vi "Settings Dialog.vi"(8 "error in (no error)":errorcluster, 11 "Settings in":T1={"Hardware Configuration"={"DAQmx Channel 1"="", "DAQmx Channel 2"="", "DAQmx Channel 3"="", "Channel 1 Name"="", "Channel 2 Name"="", "Channel 3 Name"="", "Input Config Channel 1"=-1, "Input Config Channel 2"=-1, "Input Config Channel 3"=-1, "Offset Channel 1"=0.0, "Offset Channel 2"=0.0, "Offset Channel 3"=0.0, "Scale Channel 1"=0.0, "Scale Channel 2"=0.0, "Scale Channel 3"=0.0, "Sample time"=0, "Samples per second"=0.0, "Sample mode"=0, "Samples per channel"=0, "DAQmx AI Task"="", "DAQmx Channel 4"="", "Channel 3 Name 2"="", "Input Config Channel 4"=-1, "Offset Channel 4"=0.0, "Scale Channel 4"=0.0}, "Logging Configuration"={"Log File Base Path"=path "", "TDMS File Reference"=refnum}} {"Hardware Configuration"."Input Config Channel 4" items=["Default"=-1, "RSE"=10083, "NRSE"=10078, "Differential"=10106, "Pseudodifferential"=12529]; "Hardware Configuration"."Input Config Channel 3" items=["Default"=-1, "RSE"=10083, "NRSE"=10078, "Differential"=10106, "Pseudodifferential"=12529]; "Hardware Configuration"."Input Config Channel 2" items=["Default"=-1, "RSE"=10083, "NRSE"=10078, "Differential"=10106, "Pseudodifferential"=12529]; "Hardware Configuration"."Input Config Channel 1" items=["Default"=-1, "RSE"=10083, "NRSE"=10078, "Differential"=10106, "Pseudodifferential"=12529]; "Hardware Configuration"."Sample mode" items=["Hardware Timed Single Point"=12522, "Finite Samples"=10178, "Continuous Samples"=10123]}) -> (0 "error out":errorcluster, 1 "Cancelled?":bool, 2 "UI Refresh Needed?":bool, 3 "Settings out":T1={"Hardware Configuration"={"DAQmx Channel 1"="", "DAQmx Channel 2"="", "DAQmx Channel 3"="", "Channel 1 Name"="", "Channel 2 Name"="", "Channel 3 Name"="", "Input Config Channel 1"=-1, "Input Config Channel 2"=-1, "Input Config Channel 3"=-1, "Offset Channel 1"=0.0, "Offset Channel 2"=0.0, "Offset Channel 3"=0.0, "Scale Channel 1"=0.0, "Scale Channel 2"=0.0, "Scale Channel 3"=0.0, "Sample time"=0, "Samples per second"=0.0, "Sample mode"=0, "Samples per channel"=0, "DAQmx AI Task"="", "DAQmx Channel 4"="", "Channel 3 Name 2"="", "Input Config Channel 4"=-1, "Offset Channel 4"=0.0, "Scale Channel 4"=0.0}, "Logging Configuration"={"Log File Base Path"=path "", "TDMS File Reference"=refnum}} {"Hardware Configuration"."Input Config Channel 4" items=["Default"=-1, "RSE"=10083, "NRSE"=10078, "Differential"=10106, "Pseudodifferential"=12529]; "Hardware Configuration"."Input Config Channel 3" items=["Default"=-1, "RSE"=10083, "NRSE"=10078, "Differential"=10106, "Pseudodifferential"=12529]; "Hardware Configuration"."Input Config Channel 2" items=["Default"=-1, "RSE"=10083, "NRSE"=10078, "Differential"=10106, "Pseudodifferential"=12529]; "Hardware Configuration"."Input Config Channel 1" items=["Default"=-1, "RSE"=10083, "NRSE"=10078, "Differential"=10106, "Pseudodifferential"=12529]; "Hardware Configuration"."Sample mode" items=["Hardware Timed Single Point"=12522, "Finite Samples"=10178, "Continuous Samples"=10123]})   [LabVIEW 2018, in "Settings.lvlib"]
doc: "Dialog for selecting user specified settings."
uses:
  Settings.lvlib
  Settings.ctl
  Acquisition/Hardware Configuration.ctl
  Logging/Logging Configuration.ctl
  <vilib>/Utility/xml.llb/Write to XML File(string).vi
  Acquisition/Acquisition.lvlib
  Logging/Logging.lvlib
panel:
  in  "Scale Channel 4":dbl
  in  "Offset Channel 4":dbl
  in  "Input Config Channel 4":i32(ring)=-1 items=["Default"=-1, "RSE"=10083, "NRSE"=10078, "Differential"=10106, "Pseudodifferential"=12529]
  in  "Input Config Channel 3":i32(ring)=-1 items=["Default"=-1, "RSE"=10083, "NRSE"=10078, "Differential"=10106, "Pseudodifferential"=12529]
  in  "Input Config Channel 2":i32(ring)=-1 items=["Default"=-1, "RSE"=10083, "NRSE"=10078, "Differential"=10106, "Pseudodifferential"=12529]
  in  "Input Config Channel 1":i32(ring)=-1 items=["Default"=-1, "RSE"=10083, "NRSE"=10078, "Differential"=10106, "Pseudodifferential"=12529]
  in  "Channel 4":tag="SimDev1/ai0"
  in  "Channel 4 Name":string="Battery Voltage"
  in  "Scale Channel 3":dbl
  in  "Scale Channel 2":dbl
  in  "Scale Channel 1":dbl
  in  "Offset Channel 3":dbl
  in  "Offset Channel 2":dbl
  in  "Offset Channel 1":dbl
  in  "Sample Mode":u16(ring)=10123 items=["Finite Samples"=10178, "Continuous Samples"=10123, "Hardware Timed Single Point"=12522]
  in  "Samples per channel":u32
  in  "Samples per second":dbl=1000.0
  in  "Sample time in ms":u32=10
  in  "Channel 3 Name":string="Brake torque"
  in  "Channel 2 Name":string="Battery Current"
  in  "Channel 1 Name":string="Battery Voltage"
  in  "Channel 3":tag="SimDev1/ai2"
  in  "Channel 2":tag="SimDev1/ai1"
  in  "Log File Path":path
  in  "Channel 1":tag="SimDev1/ai0"
  in  "Cancel Button":bool
  in  "OK Button":bool
  # "Non visible portion of dialog (needed for connector pane)."
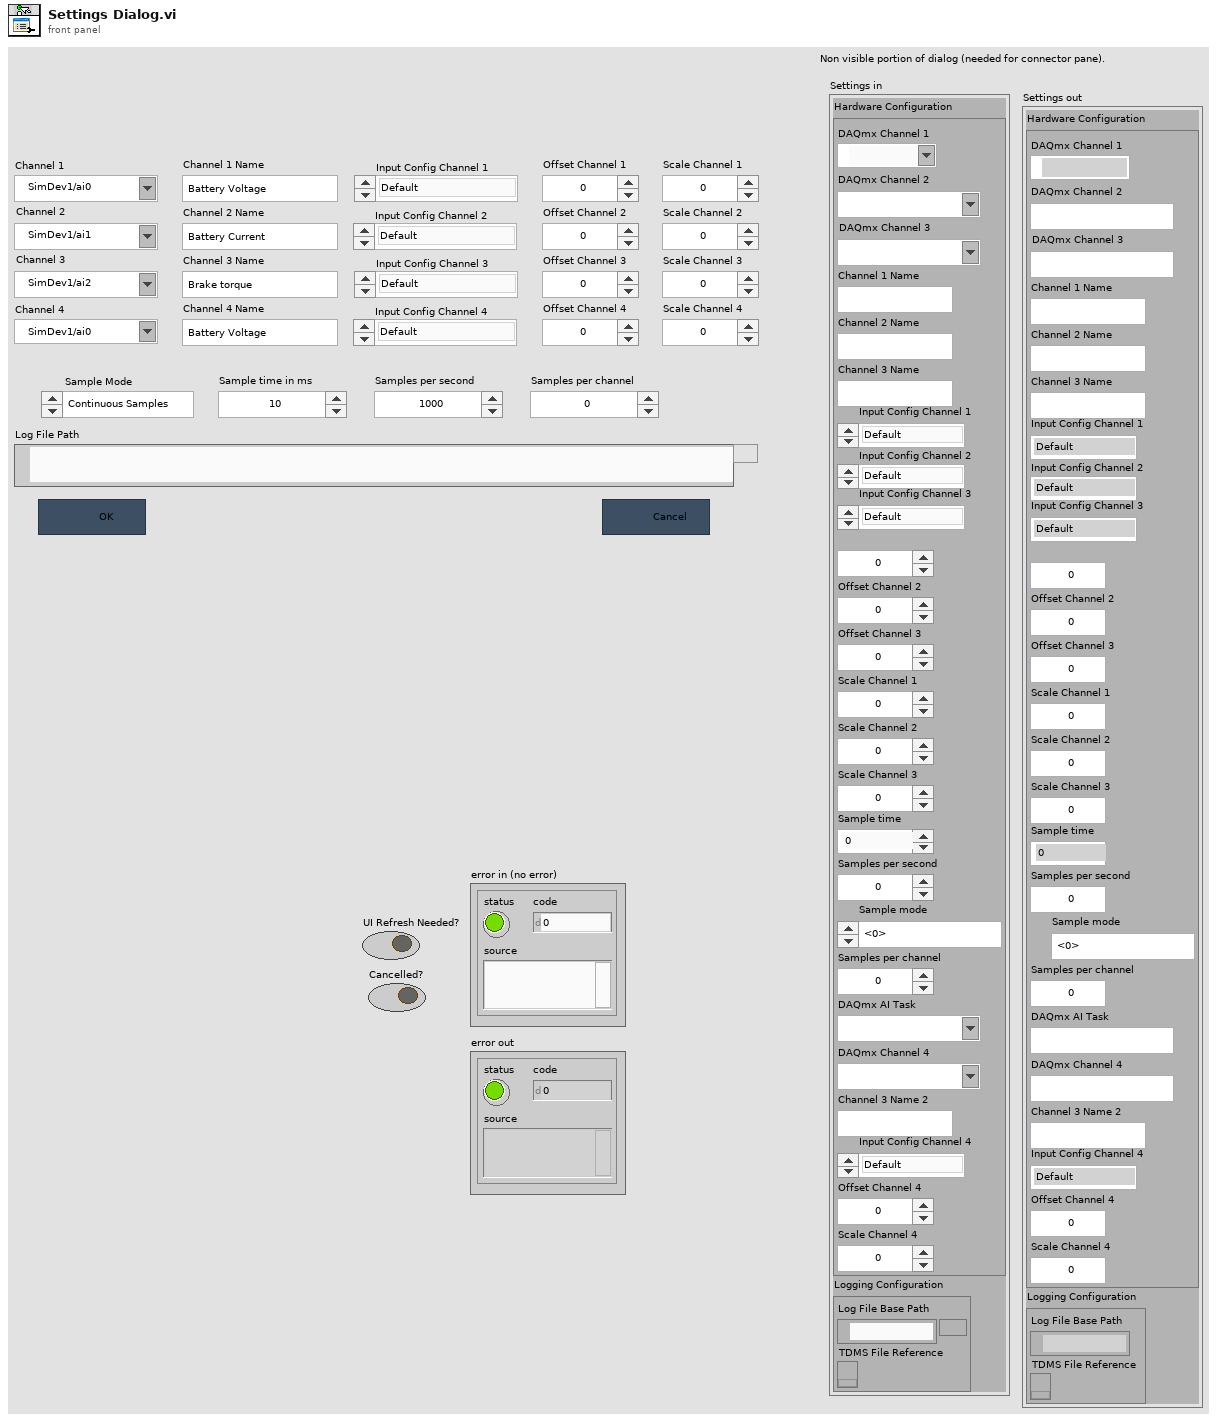
[diagram p1: front panel]
types:
  T1 = typedef "Settings.lvlib/Settings.ctl" = cluster{"Hardware Configuration":T2, "Logging Configuration":T3}
  T2 = typedef "Acquisition.lvlib/Hardware Configuration.ctl" = cluster{"DAQmx Channel 1":tag, "DAQmx Channel 2":tag, "DAQmx Channel 3":tag, "Channel 1 Name":string, "Channel 2 Name":string, "Channel 3 Name":string, "Input Config Channel 1":i32, "Input Config Channel 2":i32, "Input Config Channel 3":i32, "Offset Channel 1":dbl, "Offset Channel 2":dbl, "Offset Channel 3":dbl, "Scale Channel 1":dbl, "Scale Channel 2":dbl, "Scale Channel 3":dbl, "Sample time":u32, "Samples per second":dbl, "Sample mode":u16, "Samples per channel":i32, "DAQmx AI Task":refnum<k21>, "DAQmx Channel 4":tag, "Channel 3 Name 2":string, "Input Config Channel 4":i32, "Offset Channel 4":dbl, "Scale Channel 4":dbl}
  T3 = typedef "Logging.lvlib/Logging Configuration.ctl" = cluster{"Log File Base Path":path, "TDMS File Reference":refnum<k34>}
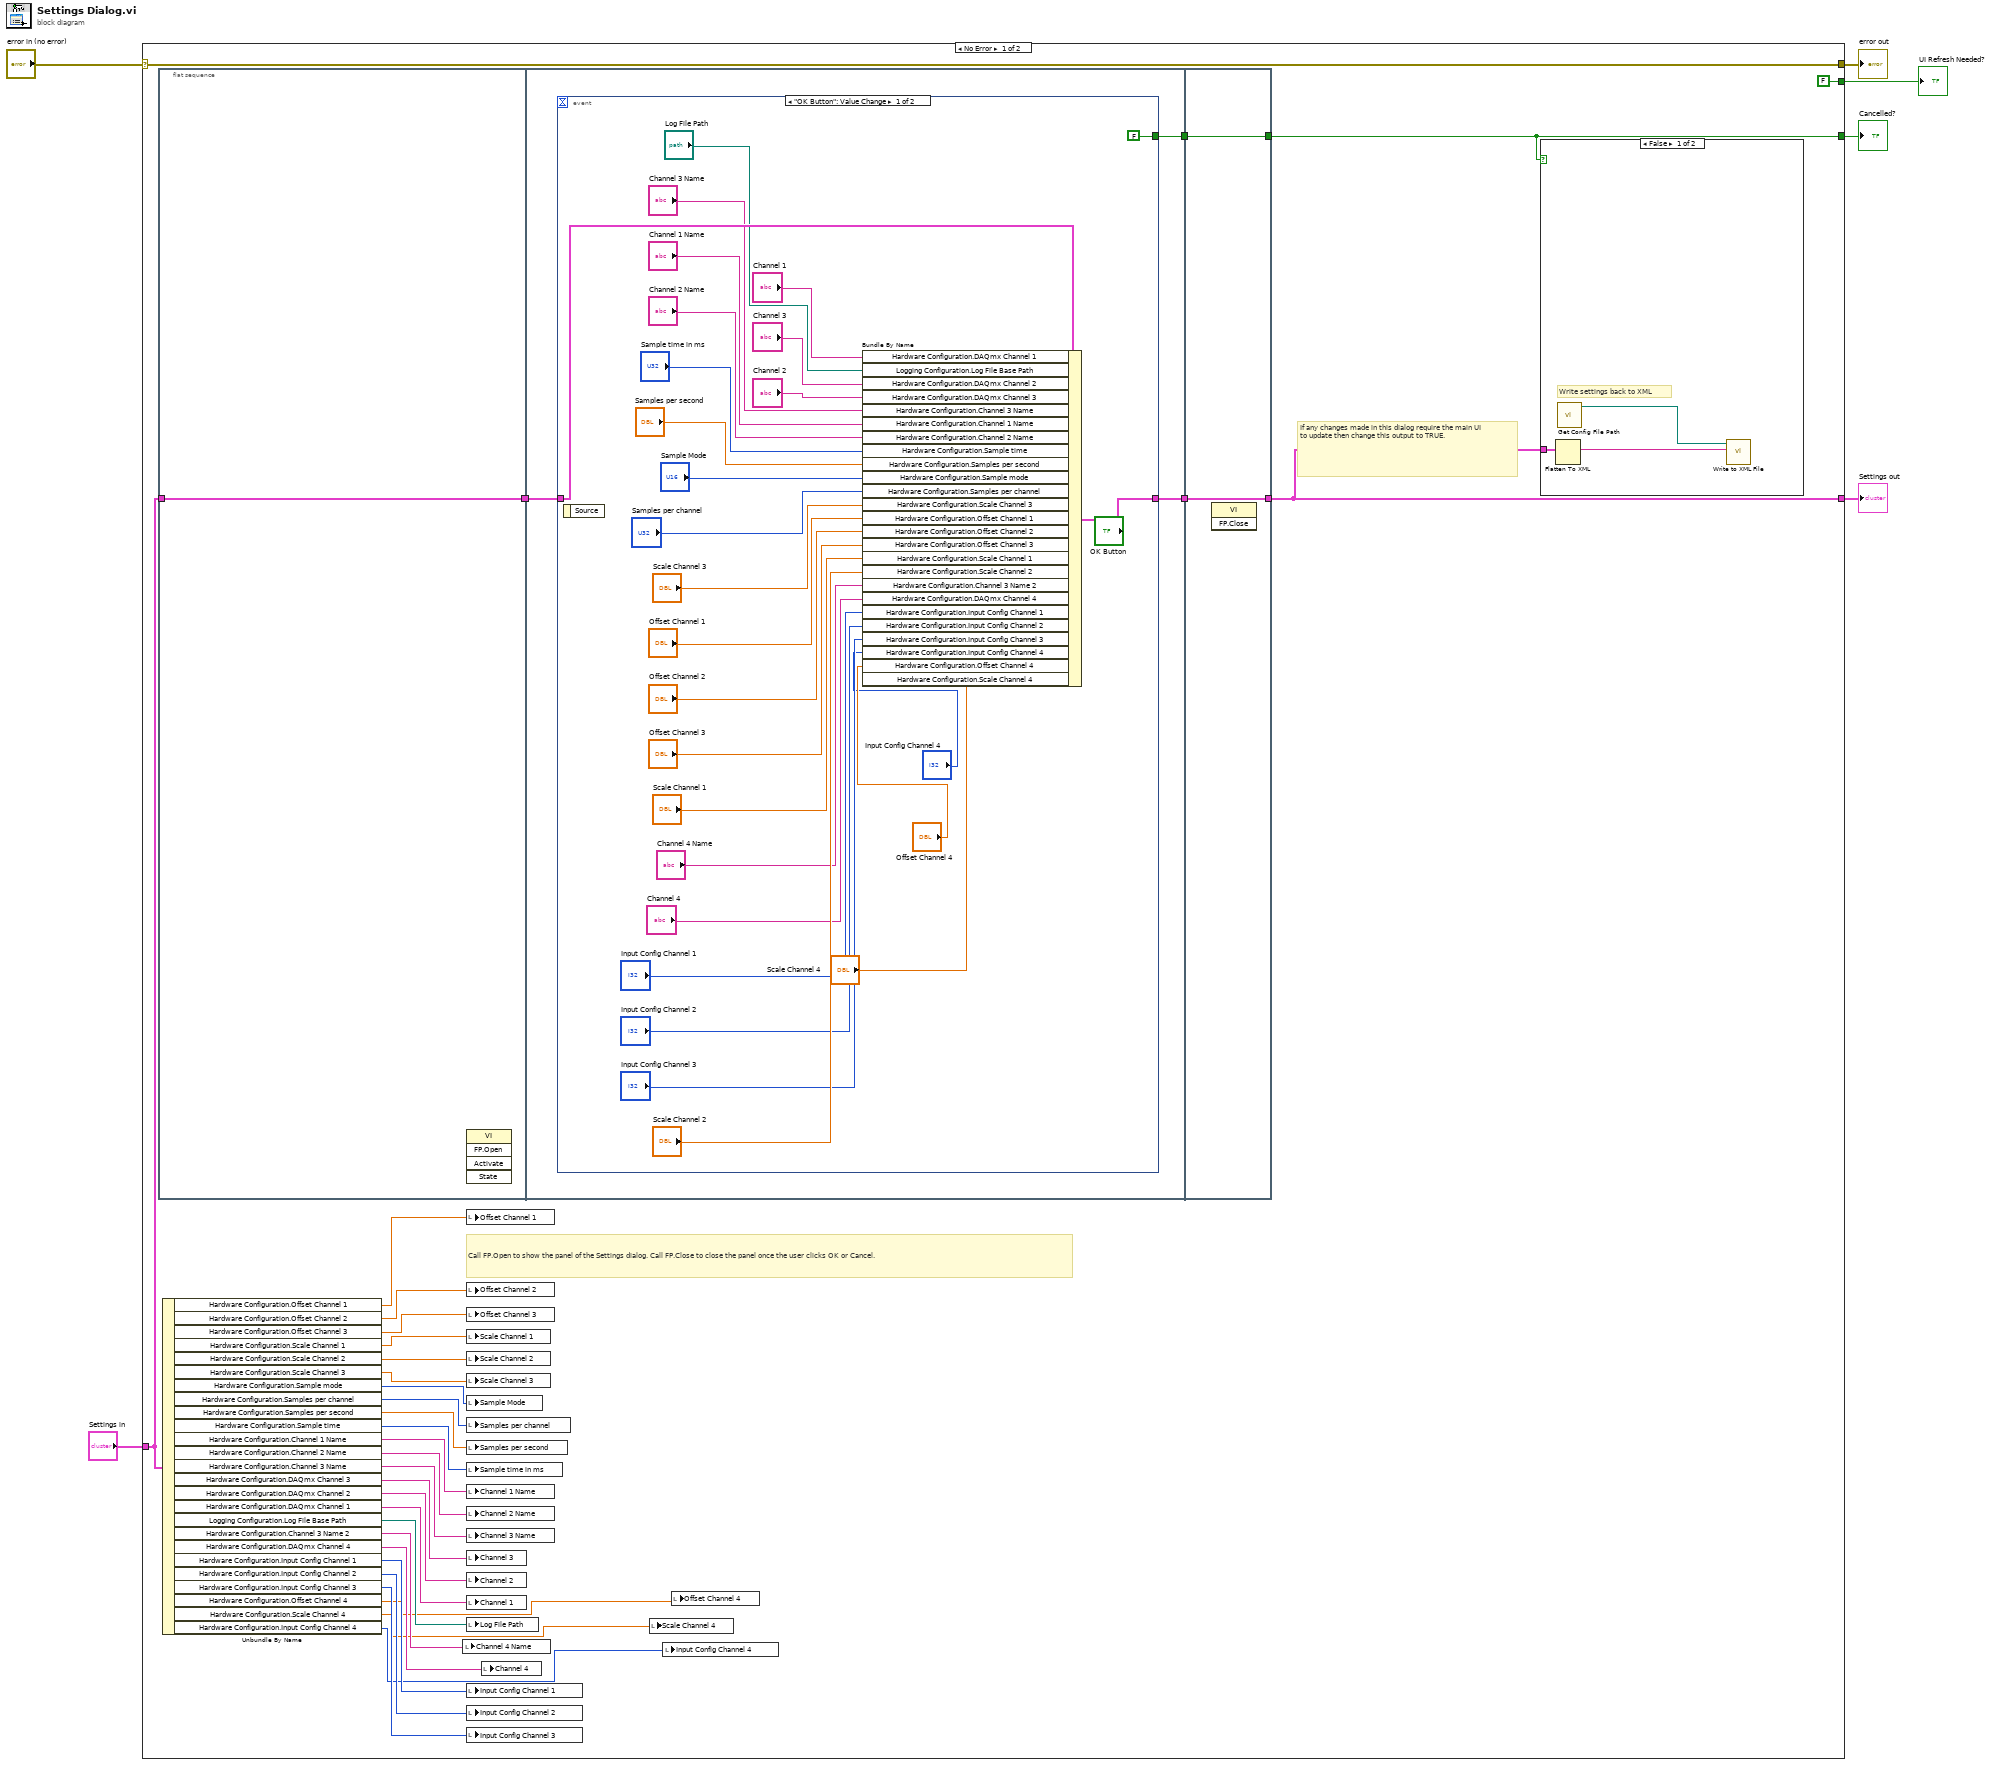
[diagram p0: block diagram]
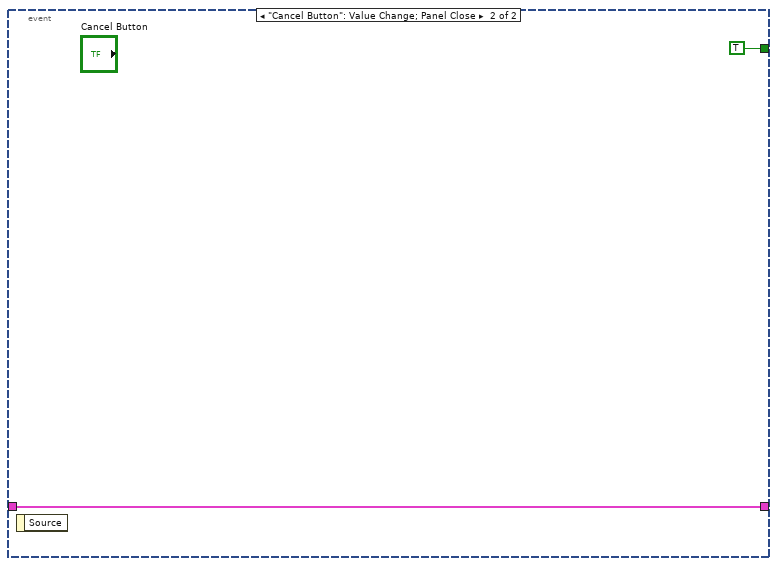
[diagram p2: hidden frame]
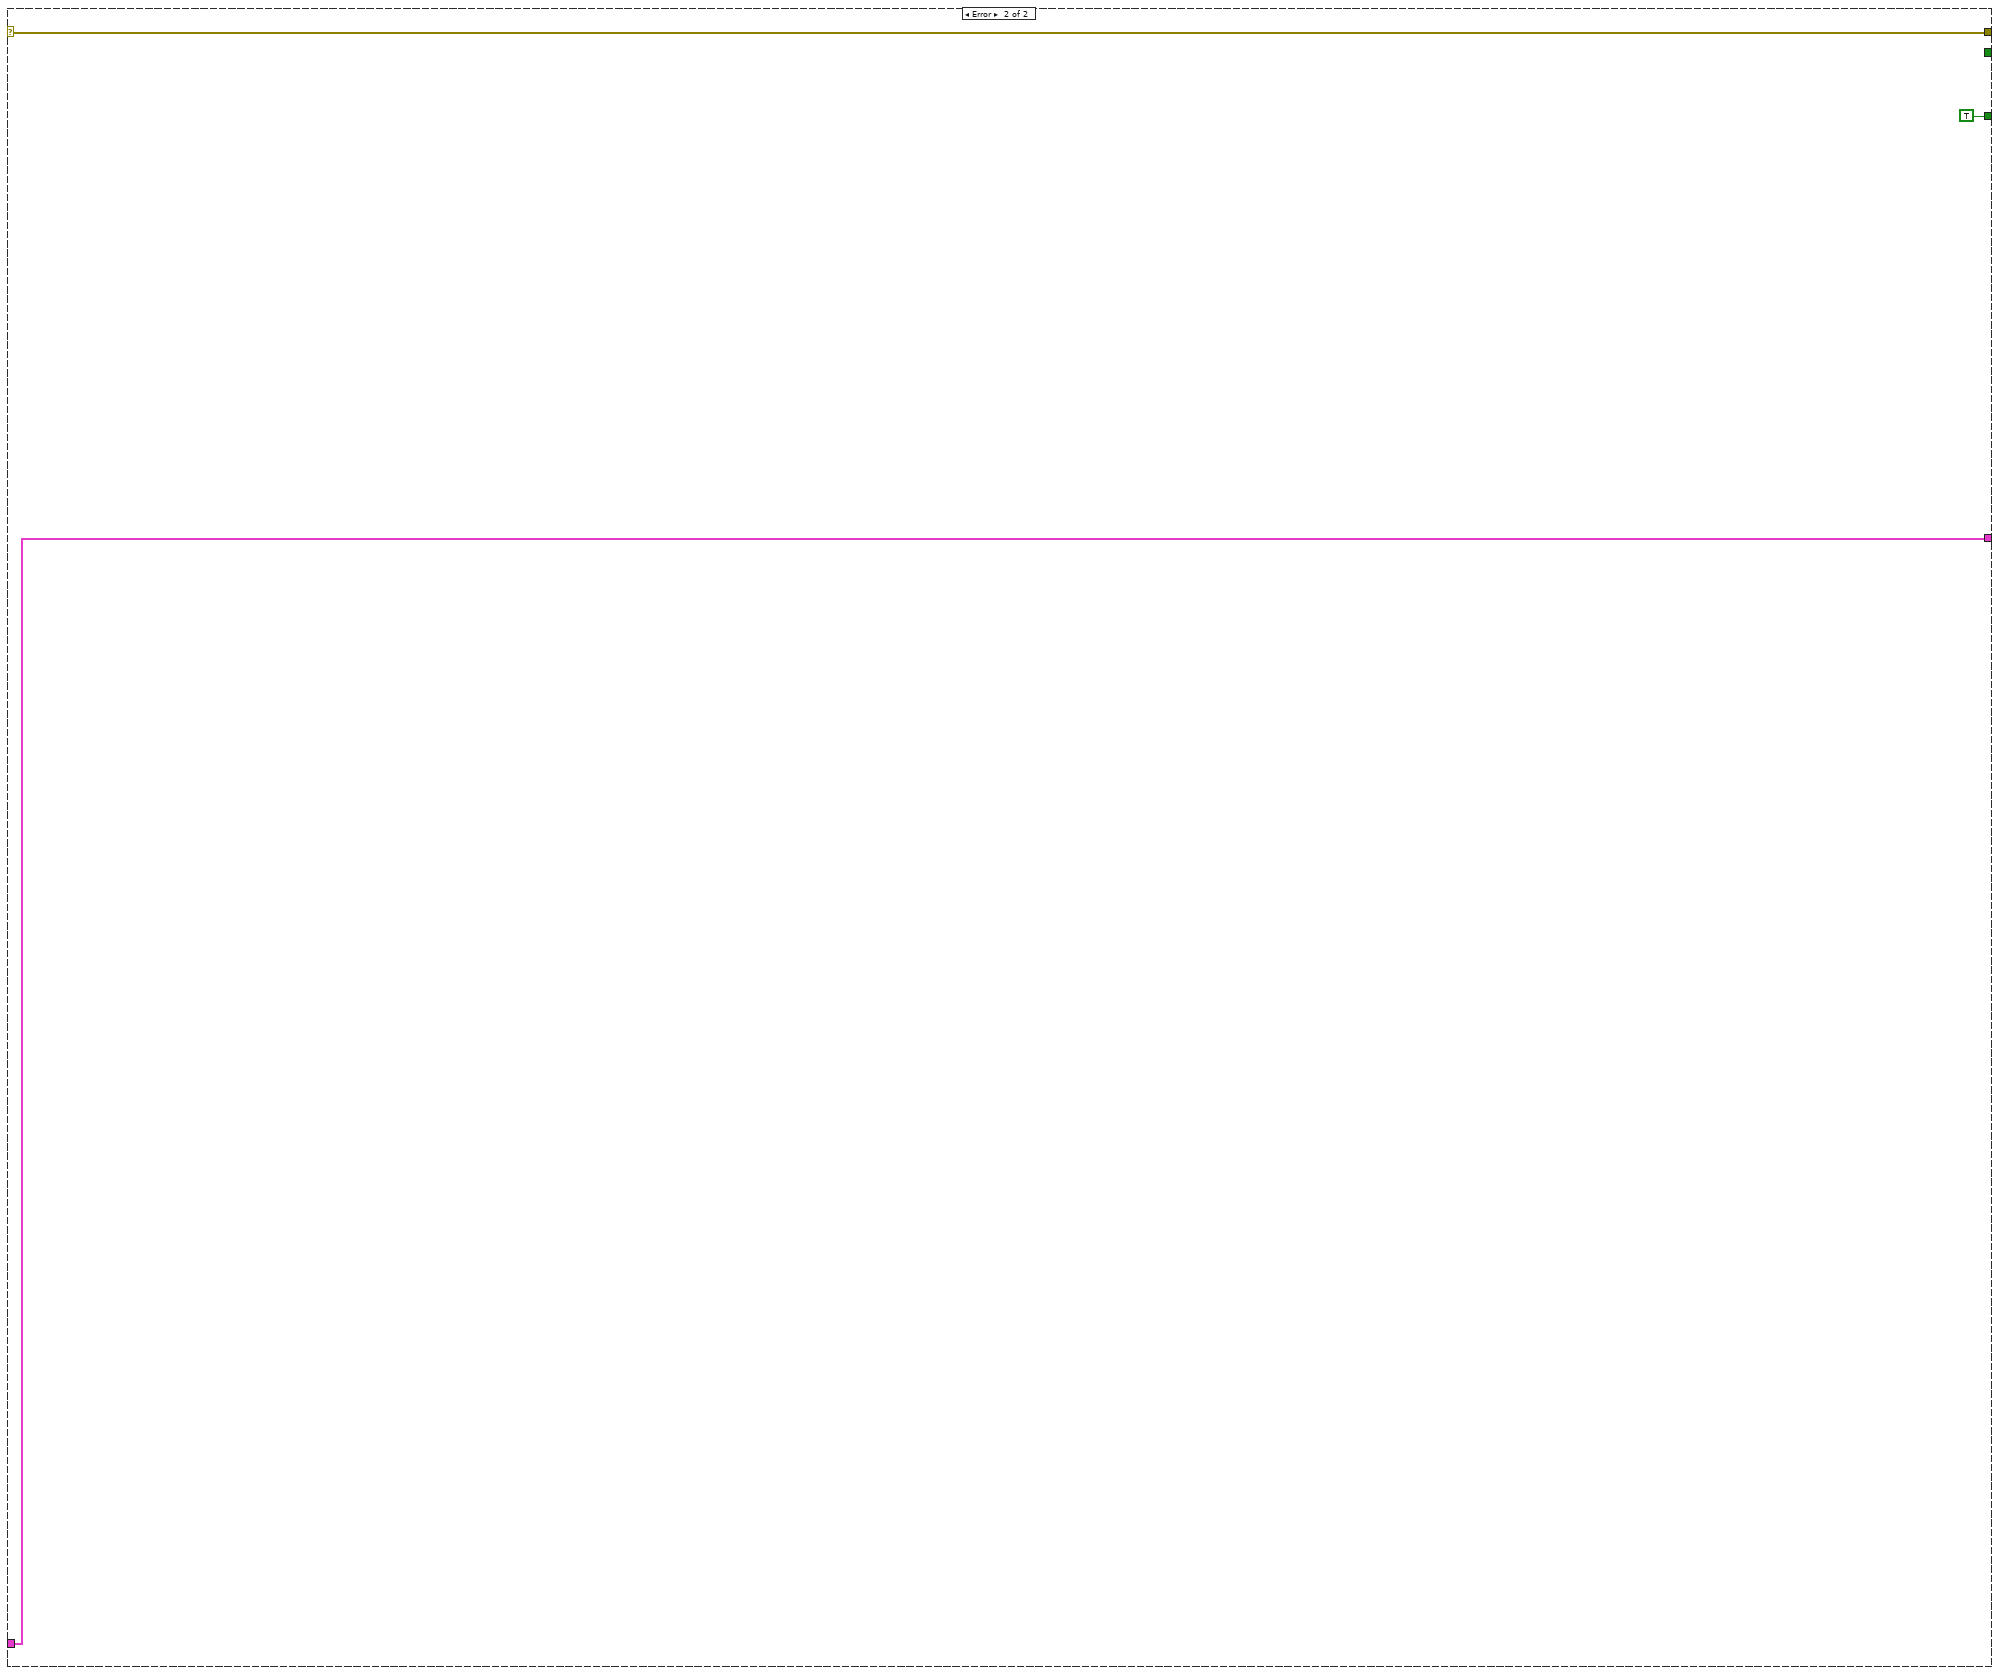
[diagram p4: hidden frame]
diagram:
  n1 = case shown="No Error" "error in (no error)" {
    selector: "error in (no error)" -> [w39 w81]
    tunnel: [w39 w81] -> w5
    tunnel: "Settings in" -> [w35 w80]
    tunnel: [w36 w80] -> w3
    tunnel: [FALSE ("UI Refresh Needed?") _] -> w2
    tunnel: [w37 TRUE ("UI Refresh Needed?")] -> w1
    frame No Error {
      # "Call FP.Open to show the panel of the Settings dialog. Call FP.Close to close the panel once the user clicks OK or Cancel."
      # "If any changes made in this dialog require the main UI to update then change this output to TRUE."
      n2 = flat-sequence {
        tunnel: w35 -> [w40]
        tunnel: [w40] -> w32
        tunnel: w32 -> [w41]
        tunnel: [w43] -> w31
        tunnel: [w42] -> w30
        tunnel: [w74] -> w36
        tunnel: [w75] -> w37
        tunnel: w31 -> [w75]
        tunnel: w30 -> [w74]
        frame #0 {
          n3 = invoke class="VI" method="FP.Open"() -> ()  [unwired: 5 in, 5 out]
        }
        frame #1 {
          n4 = event shown="[0] \"OK Button\": Value Change" {
            selector: _ -> [_ _]
            dyn-events: _ -> [_ _]
            timeout: _ -> [_ _]
            tunnel: [w69 w73] -> w42
            tunnel: w41 -> [w70 w73]
            tunnel: [FALSE ("UI Refresh Needed?") TRUE ("UI Refresh Needed?")] -> w43
            event "OK Button": Value Change {
              n5 = event-data() -> ()  [unwired: 1 in, 1 out]
              n6 = Bundle By Name(cluster=w70, "Hardware Configuration.DAQmx Channel 1"="Channel 1", "Logging Configuration.Log File Base Path"="Log File Path", "Hardware Configuration.DAQmx Channel 2"="Channel 3", "Hardware Configuration.DAQmx Channel 3"="Channel 2", "Hardware Configuration.Channel 3 Name"="Channel 3 Name", "Hardware Configuration.Channel 1 Name"="Channel 1 Name", "Hardware Configuration.Channel 2 Name"="Channel 2 Name", "Hardware Configuration.Sample time"="Sample time in ms", "Hardware Configuration.Samples per second"="Samples per second", "Hardware Configuration.Sample mode"="Sample Mode", "Hardware Configuration.Samples per channel"="Samples per channel", "Hardware Configuration.Scale Channel 3"="Scale Channel 3", "Hardware Configuration.Offset Channel 1"="Offset Channel 1", "Hardware Configuration.Offset Channel 2"="Offset Channel 2", "Hardware Configuration.Offset Channel 3"="Offset Channel 3", "Hardware Configuration.Scale Channel 1"="Scale Channel 1", "Hardware Configuration.Scale Channel 2"="Scale Channel 2", "Hardware Configuration.Channel 3 Name 2"="Channel 4 Name", "Hardware Configuration.DAQmx Channel 4"="Channel 4", "Hardware Configuration.Input Config Channel 1"="Input Config Channel 1", "Hardware Configuration.Input Config Channel 2"="Input Config Channel 2", "Hardware Configuration.Input Config Channel 3"="Input Config Channel 3", "Hardware Configuration.Input Config Channel 4"="Input Config Channel 4", "Hardware Configuration.Offset Channel 4"="Offset Channel 4", "Hardware Configuration.Scale Channel 4"="Scale Channel 4") -> (w69:T1)
            }
            event "Cancel Button": Value Change; Panel Close {
              n7 = event-data() -> ()  [unwired: 1 in, 1 out]
            }
          }
        }
        frame #2 {
          n8 = invoke class="VI" method="FP.Close"() -> ()  [unwired: 3 in, 3 out]
        }
      }
      n9 = Unbundle By Name(w35) -> ("Hardware Configuration.Offset Channel 1"=w19:dbl, "Hardware Configuration.Offset Channel 2"=w17:dbl, "Hardware Configuration.Offset Channel 3"=w20:dbl, "Hardware Configuration.Scale Channel 1"=w15:dbl, "Hardware Configuration.Scale Channel 2"=w16:dbl, "Hardware Configuration.Scale Channel 3"=w18:dbl, "Hardware Configuration.Sample mode"=w21:u16, "Hardware Configuration.Samples per channel"=w22:i32, "Hardware Configuration.Samples per second"=w23:dbl, "Hardware Configuration.Sample time"=w24:u32, "Hardware Configuration.Channel 1 Name"=w25:string, "Hardware Configuration.Channel 2 Name"=w26:string, "Hardware Configuration.Channel 3 Name"=w27:string, "Hardware Configuration.DAQmx Channel 3"=w28:tag, "Hardware Configuration.DAQmx Channel 2"=w29:tag, "Hardware Configuration.DAQmx Channel 1"=w34:tag, "Logging Configuration.Log File Base Path"=w33:path, "Hardware Configuration.Channel 3 Name 2"=w13:string, "Hardware Configuration.DAQmx Channel 4"=w14:tag, "Hardware Configuration.Input Config Channel 1"=w12:i32, "Hardware Configuration.Input Config Channel 2"=w11:i32, "Hardware Configuration.Input Config Channel 3"=w10:i32, "Hardware Configuration.Offset Channel 4"=w9:dbl, "Hardware Configuration.Scale Channel 4"=w8:dbl, "Hardware Configuration.Input Config Channel 4"=w7:i32)
      n10 = local write "Channel 4 Name"(w13) -> ()
      n11 = local write "Offset Channel 1"(w19) -> ()
      n12 = local write "Offset Channel 2"(w17) -> ()
      n13 = local write "Offset Channel 3"(w20) -> ()
      n14 = local write "Scale Channel 1"(w15) -> ()
      n15 = local write "Scale Channel 2"(w16) -> ()
      n16 = local write "Scale Channel 3"(w18) -> ()
      n17 = local write "Sample Mode"(w21) -> ()
      n18 = local write "Samples per channel"(w22) -> ()
      n19 = local write "Samples per second"(w23) -> ()
      n20 = local write "Sample time in ms"(w24) -> ()
      n21 = local write "Channel 1 Name"(w25) -> ()
      n22 = local write "Channel 2 Name"(w26) -> ()
      n23 = local write "Channel 3 Name"(w27) -> ()
      n24 = local write "Channel 3"(w28) -> ()
      n25 = local write "Channel 2"(w29) -> ()
      n26 = local write "Channel 1"(w34) -> ()
      n27 = local write "Log File Path"(w33) -> ()
      n28 = local write "Input Config Channel 1"(w12) -> ()
      n29 = local write "Input Config Channel 2"(w11) -> ()
      n30 = local write "Input Config Channel 3"(w10) -> ()
      n31 = local write "Channel 4"(w14) -> ()
      n32 = local write "Scale Channel 4"(w8) -> ()
      n33 = local write "Input Config Channel 4"(w7) -> ()
      n34 = local write "Offset Channel 4"(w9) -> ()
      n35 = case shown="False" w37 {
        tunnel: w36 -> [w77 _]
        frame False {
          # "Write settings back to XML"
          n36 = Flatten To XML(anything=w77) -> (xml string=w76:string)
          n37 = call "Get Config File Path.vi"() -> ("XML File Path"=w78:path)  [unwired: 10 in, 1 out]
          n38 = call-poly <vilib>:"Write to XML File.vi"("XML Input"=w76, "XML File Path"=w78) -> ()  [unwired: 7 in, 3 out]
        }
        frame True {
        }
      }
    }
    frame Error {
    }
  }
  "UI Refresh Needed?" <- w2
  "error out" <- w5
  "Settings out" <- w3
  "Cancelled?" <- w1
